vi "ok.vi"() -> ()   [LabVIEW 2016]
panel:
  out "Number of days":dbl
  out "last day deposite":dbl
  out "final savings":dbl
  in  "desired savings":dbl
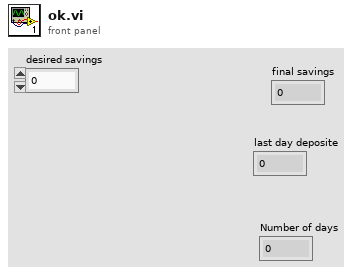
[diagram p1: front panel]
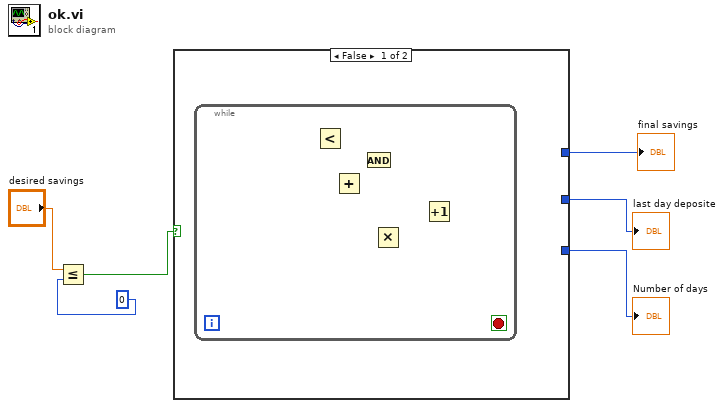
[diagram p0: block diagram]
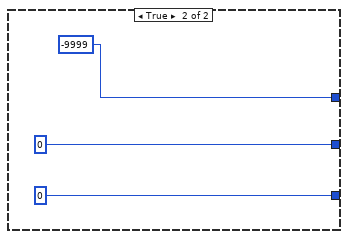
[diagram p2: hidden frame]
diagram:
  n1 = Less Or Equal?(x="desired savings", y=0) -> (x <= y?=w4:bool)
  n2 = case shown="False" w4 {
    tunnel: [_ -9999] -> w3
    tunnel: [_ 0] -> w2
    tunnel: [_ 0] -> w1
    frame False {
      n3 = while {
        stop <- _ stop-if-true
        n4 = Less?() -> ()  [unwired: 2 in, 1 out]
        n5 = Add() -> ()  [unwired: 2 in, 1 out]
        n6 = And() -> ()  [unwired: 2 in, 1 out]
        n7 = Multiply() -> ()  [unwired: 2 in, 1 out]
        n8 = Increment() -> ()  [unwired: 1 in, 1 out]
      }
    }
    frame True {
    }
  }
  "final savings" <- w3
  "last day deposite" <- w2
  "Number of days" <- w1
